vi "Init.vi"(8 "error in":errorcluster, 11 "PCAN-USB Read-Write Raw CAN Frame Strategy in":refnum<class "PCAN Base Strategy.lvclass">) -> (0 "error out":errorcluster, 3 "PCAN-USB Read-Write Raw CAN Frame Strategy out":refnum<class "PCAN Base Strategy.lvclass">)   [LabVIEW 2024, in "PCAN Base Strategy.lvclass"]
uses:
  PCAN Base Strategy.lvclass
  PCAN Base Strategy.lvclass/PCAN Base Strategy.ctl
  Source/Interfaces/IConfiguration/IConfiguration.lvclass
  <instrlib>/KDI Digital Instrumentation/API_for_PCAN_BASIC_FD/TPCANHandle.ctl
  <instrlib>/KDI Digital Instrumentation/API_for_PCAN_BASIC_FD/Error language selector.ctl
  <instrlib>/KDI Digital Instrumentation/API_for_PCAN_BASIC_FD/TPCANBaudrate.ctl
  Common-LabVIEW-Helpers/Source/NET based Helpers.lvlib
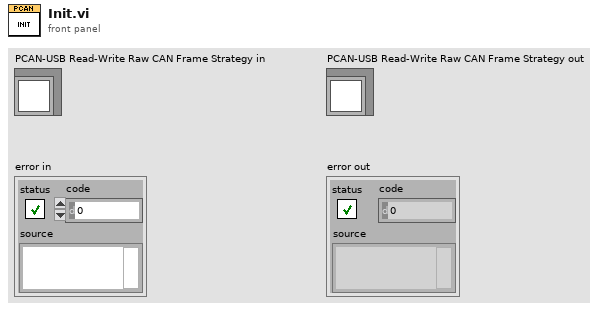
[diagram p1: front panel]
types:
  T1 = typedef "TPCANHandle.ctl" = enum16{"PCAN_NONEBUS  0x000", "PCAN_ISABUS1  0x21", "PCAN_ISABUS2  0x22", "PCAN_ISABUS3  0x23", "PCAN_ISABUS4  0x24", "PCAN_ISABUS5  0x25", "PCAN_ISABUS6  0x26", "PCAN_ISABUS7  0x27", "PCAN_ISABUS8  0x28", "PCAN_DNGBUS1  0x31", "PCAN_PCIBUS1  0x41", "PCAN_PCIBUS1  0x42", "PCAN_PCIBUS1  0x43", "PCAN_PCIBUS1  0x44", "PCAN_PCIBUS1  0x45", "PCAN_PCIBUS1  0x46", "PCAN_PCIBUS1  0x47", "PCAN_PCIBUS1  0x48", "PCAN_PCIBUS1  0x409", "PCAN_PCIBUS1  0x40A", "PCAN_PCIBUS1  0x40B", "PCAN_PCIBUS1  0x40C", "PCAN_PCIBUS1  0x40D", "PCAN_PCIBUS1  0x40E", "PCAN_PCIBUS1  0x40F", "PCAN_PCIBUS1  0x410", "PCAN_USBBUS1  0x51", "PCAN_USBBUS2  0x52", "PCAN_USBBUS3  0x53", "PCAN_USBBUS4  0x54", "PCAN_USBBUS5  0x55", "PCAN_USBBUS6  0x56", "PCAN_USBBUS7  0x57", "PCAN_USBBUS8  0x58", "PCAN_USBBUS9  0x509", "PCAN_USBBUS10  0x50A", "PCAN_USBBUS11  0x50B", "PCAN_USBBUS12  0x50C", "PCAN_USBBUS13  0x50D", "PCAN_USBBUS14  0x50E", "PCAN_USBBUS15  0x50F", "PCAN_USBBUS16  0x510", "PCAN_PCCBUS1  0x61", "PCAN_PCCBUS2  0x62", "PCAN_LANBUS1  0x801", "PCAN_LANBUS2  0x802", "PCAN_LANBUS3  0x803", "PCAN_LANBUS4  0x804", "PCAN_LANBUS5  0x805", "PCAN_LANBUS6  0x806", "PCAN_LANBUS7  0x807", "PCAN_LANBUS8  0x808", "PCAN_LANBUS9  0x809", "PCAN_LANBUS10  0x80A", "PCAN_LANBUS11  0x80B", "PCAN_LANBUS12  0x80C", "PCAN_LANBUS13  0x80D", "PCAN_LANBUS14  0x80E", "PCAN_LANBUS15  0x80F", "PCAN_LANBUS16  0x810"}
  T2 = typedef "TPCANBaudrate.ctl" = enum16{"PCAN_BAUD_1M 0x0014", "PCAN_BAUD_800K 0x0016", "PCAN_BAUD_500K 0x001C", "PCAN_BAUD_250K 0x011C", "PCAN_BAUD_125K 0x031C", "PCAN_BAUD_100K 0x432F", "PCAN_BAUD_95K 0xC34E", "PCAN_BAUD_83K 0x852B", "PCAN_BAUD_50K 0x472F", "PCAN_BAUD_47K 0x1414", "PCAN_BAUD_33K 0x8B2F", "PCAN_BAUD_20K 0x532F", "PCAN_BAUD_10K 0x672F", "PCAN_BAUD_5K 0x7F7F", "User Baudrate"}
  T3 = typedef "Error language selector.ctl" = u16
  T4 = typedef "Channel Availability.ctl" = enum16{"PCAN_CHANNEL_UNAVAILABLE", "PCAN_CHANNEL_AVAILABLE", "PCAN_CHANNEL_OCCUPIED", "PCAN_CHANNEL_PCANVIEW "}
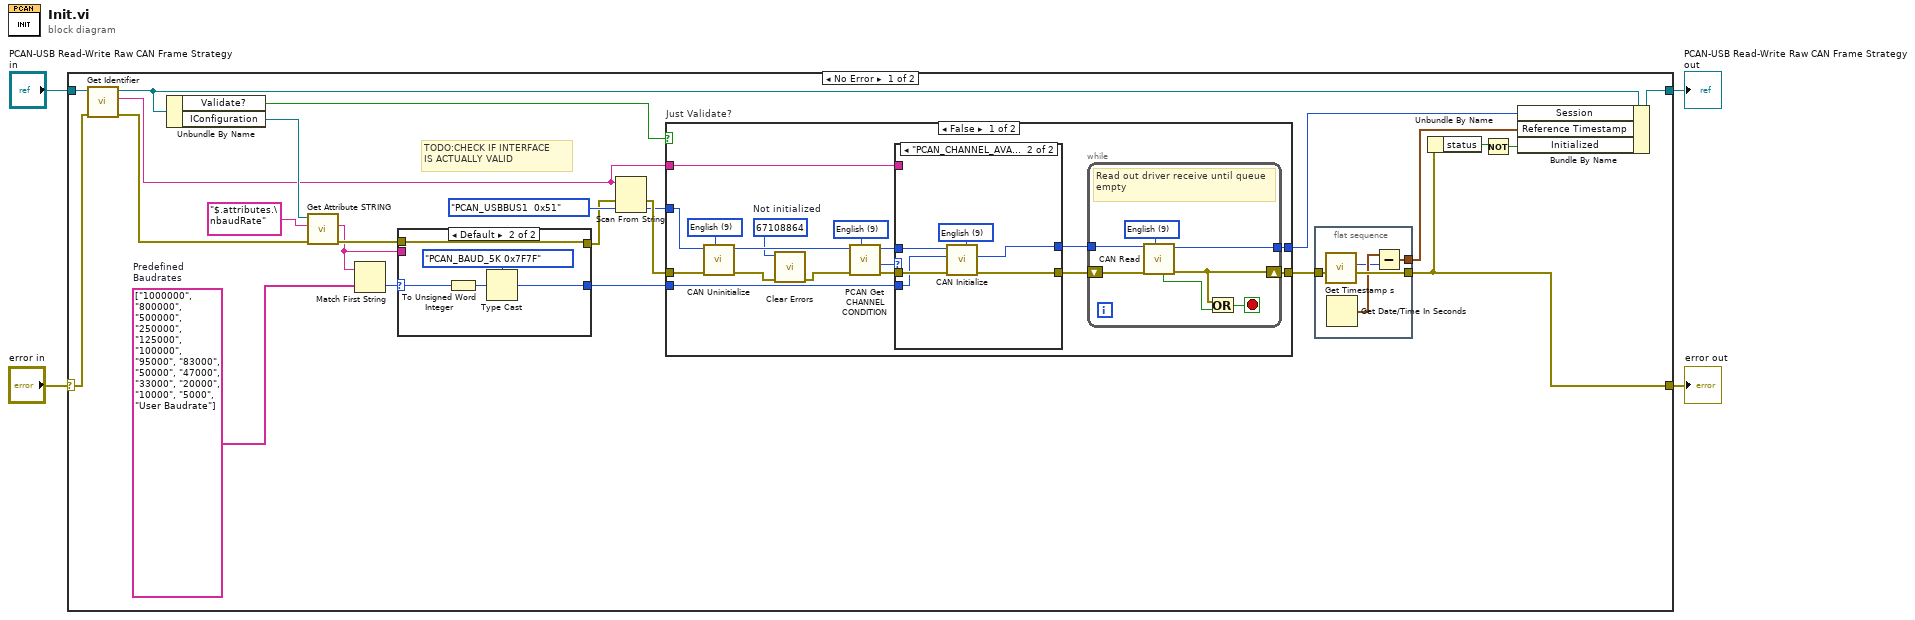
[diagram p0: block diagram]
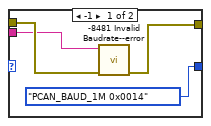
[diagram p2: hidden frame]
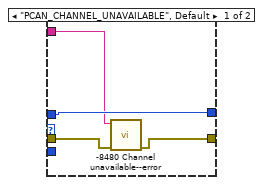
[diagram p3: hidden frame]
diagram:
  n1 = case shown="No Error" "error in" {
    selector: "error in" -> [w26 w79]
    tunnel: "PCAN-USB Read-Write Raw CAN Frame Strategy in" -> [w28 w78]
    tunnel: [w24 w78] -> w2
    tunnel: [w7 w79] -> w1
    frame No Error {
      w15 = string[] ["1000000", "800000", "500000", "250000", "125000", "100000", "95000", "83000", "50000", "47000", "33000", "20000", "10000", "5000", "User Baudrate"]  # Predefined Baudrates
      # "TODO:CHECK IF INTERFACE\nIS ACTUALLY VALID"
      n2 = call-dynamic "Get Identifier.vi"("error in"=w26, "PCAN-USB Read-Write Raw CAN Frame Strategy in"=w28) -> ("error out"=w25:errorcluster, "Instrument Identifier"=w16:string, "PCAN-USB Read-Write Raw CAN Frame Strategy out"=w23:refnum<class "PCAN Base Strategy.lvclass">)  [unwired: 7 in]
      n3 = Unbundle By Name(w23) -> ("Validate?"=w22:bool, "IConfiguration"=w27:refnum<class "IConfiguration.lvclass">)
      n4 = call-dynamic "Get Attribute STRING.vi"("error in"=w25, "Attribute"="$.attributes.\nbaudRate", "IConfiguration in"=w27) -> ("error out"=w12:errorcluster, "Value"=w10:string)  [unwired: 6 in, 1 out]
      n5 = Match First String(2:w15, 3:w10) -> (0:w14:i32)  [unwired: 1 out]
      n6 = case shown="Default" w14 {
        selector: w14 -> [_ w42]
        tunnel: [TPCANBaudrate."PCAN_BAUD_1M 0x0014" ("TPCANBaudrate") w41] -> w13
        tunnel: w12 -> [w37 w38]
        tunnel: [w36 w38] -> w11
        tunnel: w10 -> [w35 _]
        frame -1 {
          n7 = call "-8481 Invalid Baudrate--error.vi"("error in"=w37, "Baudrate"=w35) -> ("error out"=w36:errorcluster)  [unwired: 9 in]
        }
        frame Default {
          n8 = To Unsigned Word Integer(number=w42) -> (unsigned 16bit integer=w39:u16)
          n9 = Type Cast(type=TPCANBaudrate."PCAN_BAUD_5K 0x7F7F" ("TPCANBaudrate"), x=w39) -> (*(type *) &x=w41:T2)
        }
      }
      n10 = Scan From String(input string=w16, error in=w11, default 1=TPCANHandle."PCAN_USBBUS1  0x51" ("TPCANHandle")) -> (error out=w19:errorcluster, output 1=w18:T1)  [unwired: 2 in, 2 out]
      n11 = case "Just Validate?" shown="False" w22 {
        tunnel: w19 -> [w46 w77]
        tunnel: [w58 w77] -> w9
        tunnel: [w57 _] -> w17
        tunnel: w18 -> [w49 _]
        tunnel: w13 -> [w50 _]
        tunnel: w16 -> [w48 _]
        frame False {
          w44 = 67108864  # Not initialized
          w51 = T3 9 items=["System dependent", "Not available", "Not available", "Not available", "Not available", "Not available", "Not available", "Deutsch", "Not available", "English", "Español", "Not available", "Français", "Not available", "Not available", "Not available", "Italiano"] ("Language")
          w59 = T3 9 items=["System dependent", "Not available", "Not available", "Not available", "Not available", "Not available", "Not available", "Deutsch", "Not available", "English", "Español", "Not available", "Français", "Not available", "Not available", "Not available", "Italiano"] ("Language")
          n12 = call <instrlib>:"CAN Uninitialize.vi"("Language"=w59, "error in (no error)"=w46, "TPCANHandle"=w49) -> ("error out"=w45:errorcluster, "TPCANHandle out"=w47:T1)  [unwired: 6 in, 1 out]
          n13 = call <vilib>:"Clear Errors.vi"("error in (no error)"=w45, "specific error code to clear (0: all)"=w44) -> ("error out"=w43:errorcluster)  [unwired: 4 in, 1 out]
          n14 = call <instrlib>:"PCAN Get CHANNEL CONDITION.vi"("Language"=w51, "error in (no error)"=w43, "TPCANHandle"=w47) -> ("error out"=w56:errorcluster, "Channel condition"=w55:T4, "TPCANHandle out"=w54:T1)  [unwired: 6 in]
          n15 = case shown="\"PCAN_CHANNEL_AVAILABLE\"" w55 {
            tunnel: w56 -> [w62 w69]
            tunnel: [w61 w68] -> w53
            tunnel: w54 -> [w63 w67]
            tunnel: [w63 w66] -> w52
            tunnel: w50 -> [_ w64]
            tunnel: w48 -> [w60 _]
            frame "PCAN_CHANNEL_UNAVAILABLE", Default {
              n16 = call "-8480 Channel unavailable--error.vi"("error in"=w62, "Channel"=w60) -> ("error out"=w61:errorcluster)  [unwired: 9 in]
            }
            frame "PCAN_CHANNEL_AVAILABLE" {
              w65 = T3 9 items=["System dependent", "Not available", "Not available", "Not available", "Not available", "Not available", "Not available", "Deutsch", "Not available", "English", "Español", "Not available", "Français", "Not available", "Not available", "Not available", "Italiano"] ("Language")
              n17 = call <instrlib>:"CAN Initialize.vi"("Language"=w65, "error in (no error)"=w69, "TPCANBaudrate"=w64, "TPCANHandle"=w67) -> ("error out"=w68:errorcluster, "TPCANHandle_out"=w66:T1)  [unwired: 5 in, 1 out]
            }
          }
          n18 = while {
            shift-right: [w74] -> w58
            shift-left: w53 -> [w76]
            tunnel: w52 -> [w72]
            tunnel: [w71] -> w57
            stop <- w75 stop-if-true
            w70 = T3 9 items=["System dependent", "Not available", "Not available", "Not available", "Not available", "Not available", "Not available", "Deutsch", "Not available", "English", "Español", "Not available", "Français", "Not available", "Not available", "Not available", "Italiano"] ("Language")
            # "Read out driver receive until queue empty"
            n19 = call <instrlib>:"CAN Read.vi"("Language"=w70, "error in (no error)"=w76, "TPCANHandle"=w72) -> ("error out"=w74:errorcluster, "TPCANHandle out"=w71:T1, "rcv queue empty"=w73:bool)  [unwired: 4 in, 2 out]
            n20 = Or(x=w74, y=w73) -> (x .or. y?=w75:bool)
          }
        }
        frame True {
        }
      }
      n21 = flat-sequence {
        tunnel: w9 -> [w33]
        tunnel: [w32] -> w7
        tunnel: [w29] -> w8
        frame #0 {
          n22 = call "Get Timestamp s.vi"("error in"=w33) -> ("error out"=w32:errorcluster, "Timestamp"=w30:u64)  [unwired: 9 in]
          n23 = Get Date/Time In Seconds() -> (seconds since 1Jan1904=w31:timestamp)
          n24 = Subtract(x=w31, y=w30) -> (x-y=w29:timestamp)
        }
      }
      n25 = Unbundle By Name(w7) -> ("status"=w6:bool)
      n26 = Not(x=w6) -> (.not. x?=w5:bool)
      n27 = Bundle By Name(cluster=w23, "Session"=w17, "Reference Timestamp"=w8, "Initialized"=w5) -> (w24:refnum<class "PCAN Base Strategy.lvclass">)
    }
    frame Error {
    }
  }
  "error out" <- w1
  "PCAN-USB Read-Write Raw CAN Frame Strategy out" <- w2
